vi "Add To Slack Demo.vi"() -> ()   [LabVIEW 2015]
uses:
  Typedefs/Slack-User.ctl
panel:
  out "user":T1
  in  "Add Button":bool
  in  "client_secret":string="f1e341df902b360dfbc2bfcae092b542"
  in  "client_id":string="1023330033985.1045128173975"
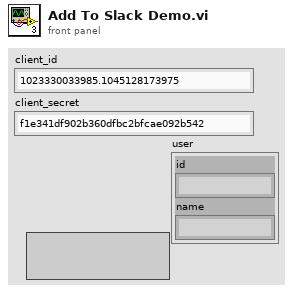
[diagram p1: front panel]
types:
  T1 = typedef "Slack-User.ctl" = cluster{"id":string, "name":string}
  T2 = typedef "Slack-Configuration.ctl" = cluster{"app_id":string, "authed_user":cluster{"id":string}, "access_token":string, "bot_user_id":string, "team":cluster{"id":string, "name":string}, "bot channel":cluster{"id":string, "name":string}, "bot_user_name":string}
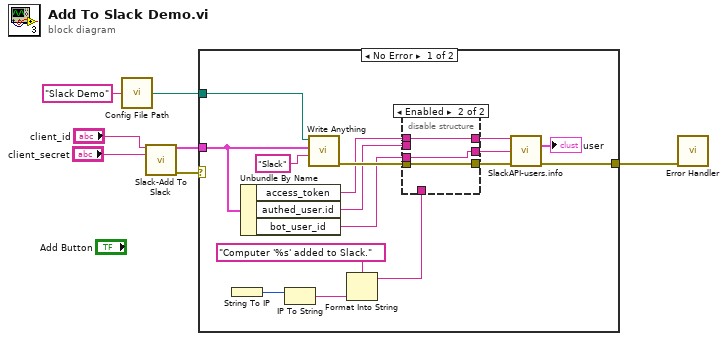
[diagram p0: block diagram]
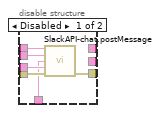
[diagram p2: hidden frame]
diagram:
  n1 = call "Config File Path.vi"("AppName"="Slack Demo") -> ("Default config file name"=w1:path)
  n2 = call "Slack-Add To Slack.vi"("client_id"="client_id", "client_secret"="client_secret") -> ("config"=w4:T2, "error out"=w5:errorcluster)  [unwired: 12 in]
  n3 = case shown="No Error" w5 {
    selector: w5 -> [_ w33]
    tunnel: w4 -> [w20 _]
    tunnel: [w11 w33] -> w3
    tunnel: w1 -> [w22 _]
    frame No Error {
      n4 = String To IP() -> (0:w16:u32)  [unwired: 1 in]
      n5 = Unbundle By Name(w20) -> ("access_token"=w19:string, "authed_user.id"=w17:string, "bot_user_id"=w18:string)
      n6 = IP To String(2:w16) -> (0:w14:string)  [unwired: 1 in]
      n7 = call "Write Anything.vi"("Section Name (Name of \"Anything\")"="Slack" ("Section Name (Name of \"Anything\")"), "Anything"=w20, "Path (dialog)"=w22) -> ("Error Out"=w21:errorcluster)  [unwired: 7 in, 1 out]
      n8 = Format Into String(format string="Computer '%s' added to Slack.", w14) -> (resulting string=w13:string)  [unwired: 2 in, 1 out]
      n9 = disable-structure shown="Enabled" {
        disable-tunnel: w21 -> [w29 w32]
        disable-tunnel: w19 -> [w28 w31]
        disable-tunnel: w18 -> [w27 w30]
        disable-tunnel: w17 -> [w26 _]
        disable-tunnel: w13 -> [w25 _]
        disable-tunnel: [w24 w32] -> w12
        disable-tunnel: [_ w31] -> w10
        disable-tunnel: [_ w30] -> w9
        frame Disabled {
          n10 = call "SlackAPI-chat.postMessage.vi"("access_token"=w28, "user ID"=w26, "message"=w25, "username"=w27, "error in (no error)"=w29) -> ("error out"=w24:errorcluster)  [unwired: 10 in]
        }
        frame Enabled {
        }
      }
      n11 = call "SlackAPI-users.info.vi"("token"=w10, "user"=w9, "error in (no error)"=w12) -> ("user"=→"user":T1, "error out"=w11:errorcluster)  [unwired: 10 in, 1 out]
    }
    frame Error {
    }
  }
  n12 = call "Error Handler.vi"("error in (no error)"=w3) -> ()  [unwired: 13 in, 2 out]
